vi "Second to millisecond.vi"(9 "Timeout":dbl=15.0) -> (1 "Timeout (ms)":i32)   [LabVIEW 2014, in "hse-db.lvlib" / "MySQL (TCP).lvlib"]
uses:
  MySQL (TCP).lvlib
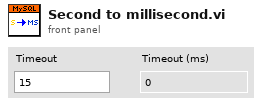
[diagram p1: front panel]
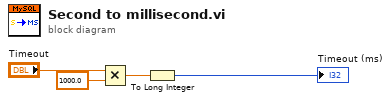
[diagram p0: block diagram]
diagram:
  n1 = Multiply(x="Timeout", y=1000.0) -> (x*y=w3:dbl)
  n2 = To Long Integer(number=w3) -> (32bit integer=→"Timeout (ms)":i32)
